vi "Set Route Parameter.vi"(6 "Connected?":bool, 8 "error in (no error)":errorcluster, 9 "Output Index":i32, 10 "Input Index":i32, 11 "VoiceMeeterRemote in":refnum<class "VoiceMeeterRemote.lvclass">) -> (0 "error out":errorcluster, 2 "Parameter Name":string, 3 "VoiceMeeterRemote out":refnum<class "VoiceMeeterRemote.lvclass">)   [LabVIEW 2022 SP3, in "VoiceMeeterRemote.lvlib" / "VoiceMeeterRemote.lvclass"]
doc: "Controls the routing of the specified input index to the specified output index. If <b>Connected?</b> is true, then audio from the input will be played on the output."
uses:
  VoiceMeeterRemote.lvclass
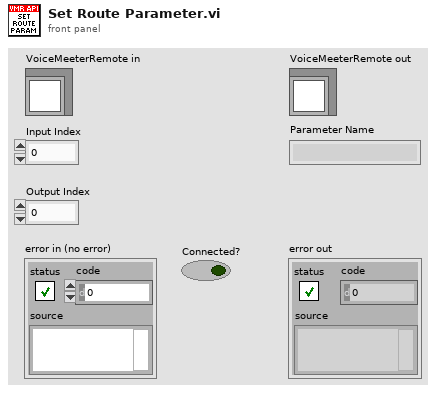
[diagram p1: front panel]
types:
  T1 = typedef "VoiceMeeterRemote.lvlib/Voicemeeter Type.ctl" = enum16{"Unknown", "Voicemeeter", "Banana", "Potato", "Potato x64"}
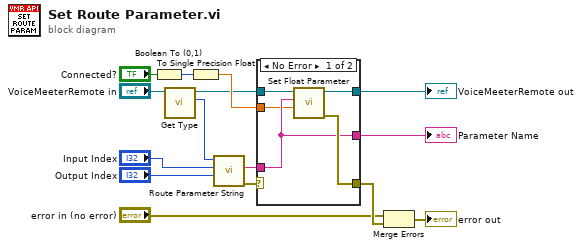
[diagram p0: block diagram]
diagram:
  n1 = Boolean To (0,1)(Boolean="Connected?") -> (0, 1=w8:i16)
  n2 = call "Get Type.vi"("VoiceMeeterRemote in"="VoiceMeeterRemote in") -> ("Type"=w5:T1, "VoiceMeeterRemote out"=w6:refnum<class "VoiceMeeterRemote.lvclass">)  [unwired: 8 in, 1 out]
  n3 = To Single Precision Float(number=w8) -> (single precision float=w7:sgl)
  n4 = call "Route Parameter String.vi"("Output Index"="Output Index", "Input Index"="Input Index", "Voicemeeter Type"=w5) -> ("error out"=w1:errorcluster, "Route Parameter String"=w2:string)  [unwired: 7 in]
  n5 = case shown="No Error" w1 {
    selector: w1 -> [_ w21]
    tunnel: w6 -> [w19 w22]
    tunnel: w2 -> [w17 _]
    tunnel: [w18 w22] -> w13
    tunnel: [w17 _] -> w9
    tunnel: [w20 w21] -> w15
    tunnel: w7 -> [w16 _]
    frame No Error {
      n6 = call "Set Float Parameter.vi"("Value"=w16, "Parameter Name"=w17, "VoiceMeeterRemote in"=w19) -> ("error out"=w20:errorcluster, "VoiceMeeterRemote out"=w18:refnum<class "VoiceMeeterRemote.lvclass">)  [unwired: 7 in]
    }
    frame Error {
    }
  }
  "VoiceMeeterRemote out" <- w13
  "Parameter Name" <- w9
  n7 = Merge Errors("error in (no error)", w15) -> (→"error out":errorcluster)
